vi "ellipse parameters from points fourier.vi"(9 "Phi":dbl[](array[numeric]), 10 "Y":dbl[](array[numeric]), 11 "X":dbl[](array[numeric])) -> (3 "ellipse parameters":T1)   [LabVIEW 2017]
panel:
  out "signed area surveyor":dbl
  out "signed area ellipse fit":dbl
  out "signed minor axis":dbl
  out "unsigned minor axis":dbl
  out "major axis":dbl
  out "major axis angle":dbl
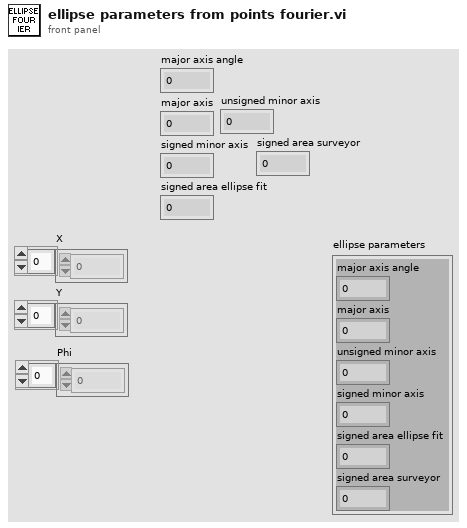
[diagram p1: front panel]
types:
  T1 = cluster{"major axis angle":dbl, "major axis":dbl, "unsigned minor axis":dbl, "signed minor axis":dbl, "signed area ellipse fit":dbl, "signed area surveyor":dbl}
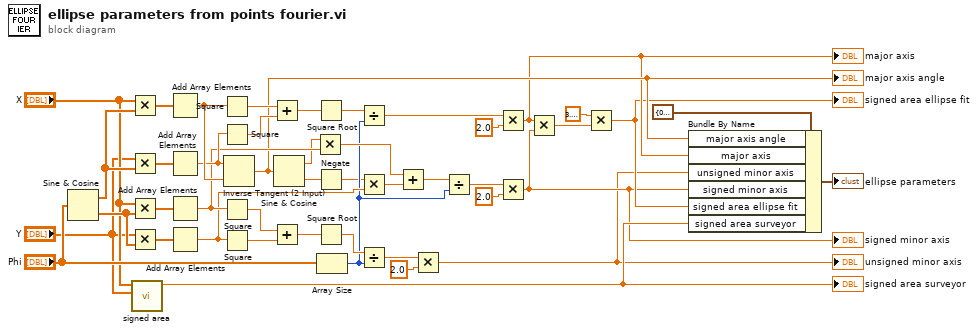
[diagram p0: block diagram]
diagram:
  n1 = Sine & Cosine(0:"Phi") -> (1:w44:dbl[], 2:w30:dbl[])
  n2 = Multiply(x="X", y=w44) -> (x*y=w43:dbl[])
  n3 = Multiply(x="Y", y=w44) -> (x*y=w42:dbl[])
  n4 = Multiply(x="X", y=w30) -> (x*y=w32:dbl[])
  n5 = Multiply(x="Y", y=w30) -> (x*y=w31:dbl[])
  n6 = call "signed area.vi"("Y"="Y", "X"="X") -> ("signed area"=w7:dbl)  [unwired: 9 in]
  "signed area surveyor" <- w7
  n7 = Add Array Elements(numeric array=w43) -> (sum=w41:dbl)
  n8 = Add Array Elements(numeric array=w42) -> (sum=w40:dbl)
  n9 = Add Array Elements(numeric array=w32) -> (sum=w21:dbl)
  n10 = Add Array Elements(numeric array=w31) -> (sum=w18:dbl)
  n11 = Square(x=w41) -> (x^2=w39:dbl)
  n12 = Square(x=w40) -> (x^2=w38:dbl)
  n13 = Square(x=w21) -> (x^2=w29:dbl)
  n14 = Square(x=w18) -> (x^2=w28:dbl)
  n15 = Inverse Tangent (2 Input)(1:w41, 2:w40) -> (0:w6:dbl)
  "major axis angle" <- w6
  n16 = Add(x=w39, y=w38) -> (x+y=w36:dbl)
  n17 = Add(x=w29, y=w28) -> (x+y=w27:dbl)
  n18 = Sine & Cosine(0:w6) -> (1:w20:dbl, 2:w19:dbl)
  n19 = Multiply(x=w20, y=w21) -> (x*y=w16:dbl)
  n20 = Square Root(x=w36) -> (sqrt(x)=w35:dbl)
  n21 = Negate(x=w19) -> (-x=w1:dbl)
  n22 = Square Root(x=w27) -> (sqrt(x)=w26:dbl)
  n23 = Array Size(array="Phi") -> (size(s)=w13:i32)
  n24 = Divide(x=w35, y=w13) -> (x/y=w34:dbl)
  n25 = Multiply(x=w1, y=w18) -> (x*y=w17:dbl)
  n26 = Divide(x=w26, y=w13) -> (x/y=w25:dbl)
  n27 = Add(x=w16, y=w17) -> (x+y=w12:dbl)
  n28 = Multiply(x=w25, y=2.0) -> (x*y=w2:dbl)
  "unsigned minor axis" <- w2
  n29 = Divide(x=w12, y=w13) -> (x/y=w15:dbl)
  n30 = Multiply(x=w34, y=2.0) -> (x*y=w5:dbl)
  "major axis" <- w5
  n31 = Multiply(x=w15, y=2.0) -> (x*y=w3:dbl)
  "signed minor axis" <- w3
  n32 = Multiply(x=w5, y=w3) -> (x*y=w11:dbl)
  n33 = Multiply(x=3.141592653589793, y=w11) -> (x*y=w4:dbl)
  "signed area ellipse fit" <- w4
  n34 = Bundle By Name(cluster=T1 {"major axis angle"=0.0, "major axis"=0.0, "unsigned minor axis"=0.0, "signed minor axis"=0.0, "signed area ellipse fit"=0.0, "signed area surveyor"=0.0} ("Cluster"), "major axis angle"=w6, "major axis"=w5, "unsigned minor axis"=w2, "signed minor axis"=w3, "signed area ellipse fit"=w4, "signed area surveyor"=w7) -> (→"ellipse parameters":T1)
